vi "Test Helper Loop Log Helper Loop Error.vi"(8 "error in (no error)":errorcluster, 11 "Helper Loop Test In":refnum<class "Helper Loop Test.lvclass">) -> (0 "error out":errorcluster, 3 "Helper Loop Test Out":refnum<class "Helper Loop Test.lvclass">)   [LabVIEW 2020, in "Helper Loop Test.lvclass"]
uses:
  Helper Loop Test.lvclass
  C:/Program Files (x86)/National Instruments/LabVIEW 2020/vi.lib/Astemes/LUnit/Test Case.lvclass
  source/Framework Test Suite/Mock Process/Mock Process.lvclass
  C:/Git/astemes-triarc-framework/source/Framework/Process/Process.lvclass
  source/Framework Test Suite/Mock Log Handler/Mock Log Handler.lvclass
  C:/Git/astemes-triarc-framework/source/Framework/Logging/Logging.lvclass
  source/Framework/Process/Process.lvclass/Process.ctl
  <vilib>/Astemes/LUnit/Test Case.lvclass/Test Case.ctl
  b4912422-9a16-4525-859a-dee64b9b2a4a.vi
  source/Framework/Process/Public/Lifecycle/Get Lifecycle State.vi
  source/Framework/Process/Protected/Messaging/Send Message.vi
  source/Framework/Process/Private/SubVIs/Wait for finish.vi
  source/Framework/Process/Private/SubVIs/Set Lifecycle State.vi
  <vilib>/Astemes/LUnit/Palette/Pass.vi
  <vilib>/Astemes/LUnit/Palette/Fail.vi
  <vilib>/Astemes/LUnit/Compare Variants.vi
  <vilib>/Astemes/LUnit/Describe Comparison.vi
  <vilib>/Astemes/LUnit/Set Assertion Type.vi
  <vilib>/Utility/error.llb/Clear Errors.vi
  source/Framework/Process/Private/SubVIs/Handle Debug Data.vi
  <vilib>/Astemes/LUnit/Add test result.vi
  <vilib>/Astemes/LUnit/Variant to string.vi
  source/Framework/Logging/Log Debug.vi
  <vilib>/AdvancedString/1D String Array to Delimited String.vi
  <vilib>/Utility/High Resolution Relative Seconds.vi
  <vilib>/Astemes/LUnit/LUnit Record Assertion Result.vi
  <vilib>/Astemes/LUnit/LUnit Aggregate Assertion Results.vi
  <vilib>/Astemes/LUnit/Method Result/LUnit Merge Status.vi
  <vilib>/Astemes/LUnit/LUnit Concatenate result strings.vi
  <vilib>/Utility/error.llb/Error Cluster From Error Code.vi
  source/Framework/Process/Public/Read Name.vi
  <vilib>/Utility/Data Type/Get Type Information.vi
  <vilib>/Utility/LVClass/Get LV Class Name.vi
  source/Framework/Process/Process.lvclass
  Helper Loop Test.lvclass/Helper Loop Test.ctl
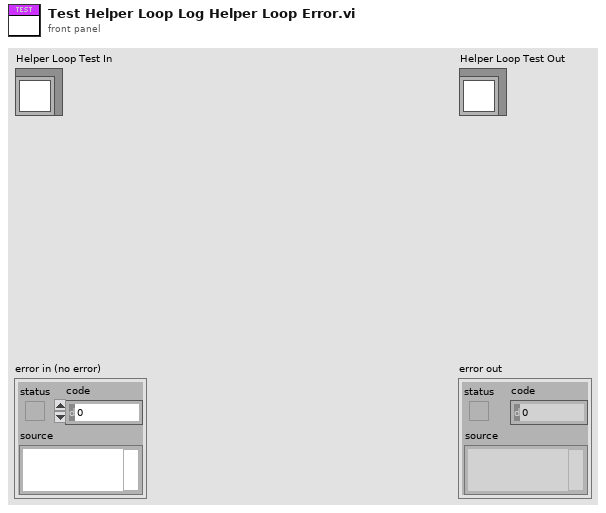
[diagram p1: front panel]
types:
  T1 = typedef "Mock Log Handler.lvclass/Log Entry.ctl" = cluster{"Level":string, "Source":string, "Message":string}
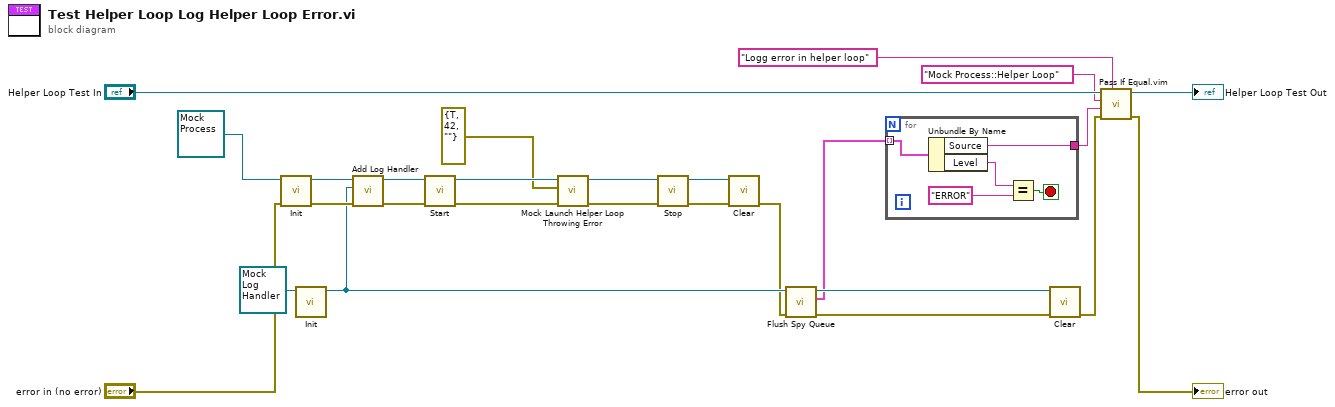
[diagram p0: block diagram]
diagram:
  n1 = call-dynamic "Init.vi"("error in (no error)"="error in (no error)", "Mock Process In"=refnum<class "Mock Process.lvclass"> refnum) -> ("error out"=w26:errorcluster, "Mock Process Out"=w13:refnum<class "Mock Process.lvclass">)  [unwired: 8 in]
  n2 = call-dynamic "Init.vi"("Mock Log Handler In"=refnum<class "Mock Log Handler.lvclass"> refnum) -> ("Mock Log Handler Out"=w10:refnum<class "Mock Log Handler.lvclass">)  [unwired: 9 in, 1 out]
  n3 = call "Add Log Handler.vi"("error in (no error)"=w26, "Log Handler"=w10, "Process In"=w13) -> ("error out"=w14:errorcluster, "Process Out"=w12:refnum<class "Mock Process.lvclass">)  [unwired: 7 in]
  n4 = call "Start.vi"("error in (no error)"=w14, "Process In"=w12) -> ("error out"=w24:errorcluster, "Process Out"=w25:refnum<class "Mock Process.lvclass">)  [unwired: 7 in, 1 out]
  n5 = call "Mock Launch Helper Loop Throwing Error.vi"("error in (no error)"=w24, "Error message"=errorcluster {"status"=TRUE, "code"=42, "source"=""}, "Mock Process in"=w25) -> ("error out"=w9:errorcluster, "Mock Process out"=w23:refnum<class "Mock Process.lvclass">)  [unwired: 7 in]
  n6 = call "Stop.vi"("error in (no error)"=w9, "Process In"=w23) -> ("error out"=w22:errorcluster, "Process Out"=w15:refnum<class "Mock Process.lvclass">)  [unwired: 7 in, 1 out]
  n7 = call-dynamic "Clear.vi"("error in (no error)"=w22, "Mock Process In"=w15) -> ("error out"=w8:errorcluster)  [unwired: 9 in]
  n8 = call "Flush Spy Queue.vi"("error in (no error)"=w8, "Mock Log Handler in"=w10) -> ("error out"=w6:errorcluster, "remaining elements"=w3:T1[], "Mock Log Handler out"=w7:refnum<class "Mock Log Handler.lvclass">)  [unwired: 7 in]
  n9 = for {
    tunnel: w3 -> [w31] mode=indexing
    tunnel: [w27] -> w2
    stop <- w30 stop-if-true
    n10 = Unbundle By Name(w31) -> ("Source"=w27:string, "Level"=w28:string)
    n11 = Equal?(x=w28, y="ERROR") -> (x = y?=w30:bool)
  }
  n12 = call-dynamic "Clear.vi"("error in (no error)"=w6, "Mock Log Handler In"=w7) -> ("error out"=w5:errorcluster)  [unwired: 9 in]
  n13 = call "Pass If Equal.vim"("Description"="Logg error in helper loop", "error in (no error)"=w5, "Actual"=w2, "Expected"="Mock Process::Helper Loop", "LUnit Test Case In"="Helper Loop Test In") -> ("error out"=→"error out":errorcluster, "LUnit Test Case Out"=→"Helper Loop Test Out":refnum<class "Helper Loop Test.lvclass">)  [unwired: 5 in]
